vi "2L12-OBS_R(t).vi"(11 "N(t)":dbl[](array[numeric])) -> (3 "R(t)":dbl[](array[numeric]))   [LabVIEW 2010, in "lv_02.lvlib"]
uses:
  lv_02.lvlib
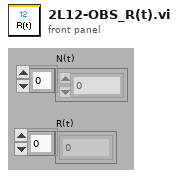
[diagram p1: front panel]
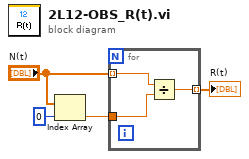
[diagram p0: block diagram]
diagram:
  n1 = Index Array(array="N(t)", index=0 ("indice")) -> (element=w2:dbl)
  n2 = for {
    tunnel: "N(t)" -> [w7] mode=indexing
    tunnel: w2 -> [w6]
    tunnel: [w5] -> w1 mode=indexing
    n3 = Divide(x=w7, y=w6) -> (x/y=w5:dbl)
  }
  "R(t)" <- w1
